vi "dfd_Convert Waveform Graph to XY Graph.vi"(10 "waveforms":cluster{"f0":dbl, "df":dbl, "values":dbl[]}[](array[cluster])) -> (2 "XY graphs":cluster{dbl[], "values":dbl[]}[](array[cluster]))   [LabVIEW 2017, in "NI_DigFilter_FilterBank.lvlib"]
uses:
  <vilib>/addons/Digital Filter Design/NI_DigFilter_FilterBank.lvlib
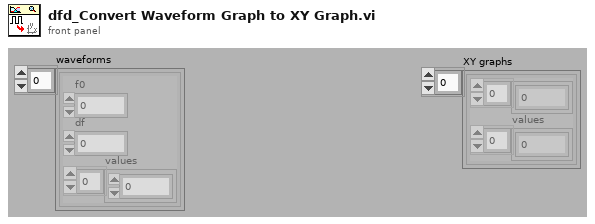
[diagram p1: front panel]
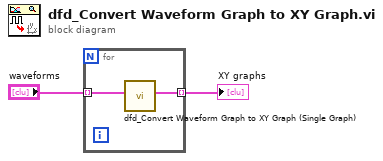
[diagram p0: block diagram]
diagram:
  n1 = for {
    tunnel: "waveforms" -> [w4] mode=indexing
    tunnel: [w3] -> w2 mode=indexing
    n2 = call <vilib>:"dfd_Convert Waveform Graph to XY Graph (Single Graph).vi"("waveform"=w4) -> ("XY graph"=w3:cluster{dbl[], "values":dbl[]})  [unwired: 10 in]
  }
  "XY graphs" <- w2
